vi "AuMT8852B Initial Carrier Extended Results Query.vi"(7 "Stage":T1(ring), 8 "error in (no error)":errorcluster, 11 "VISA session":refnum<visa-resource-name>) -> (0 "error out":errorcluster, 2 "error code":i32, 3 "VISA session out":refnum<visa-resource-name>, 4 "Results":T2 {"Max negative offset (kHz)" format="%.2f"; "Max positive offset (kHz)" format="%.2f"; "Test average offset (kHz)" format="%.2f"})   [LabVIEW 2017]
doc: "Anritsu MT8852B Bluetooth Tester\n\nReturns the results of the Initial Carrier test.\n\nINPUTS\nStage - results of the individual hopping stages of the test.\n\nOUTPUTS\nResults - measurements made during the test."
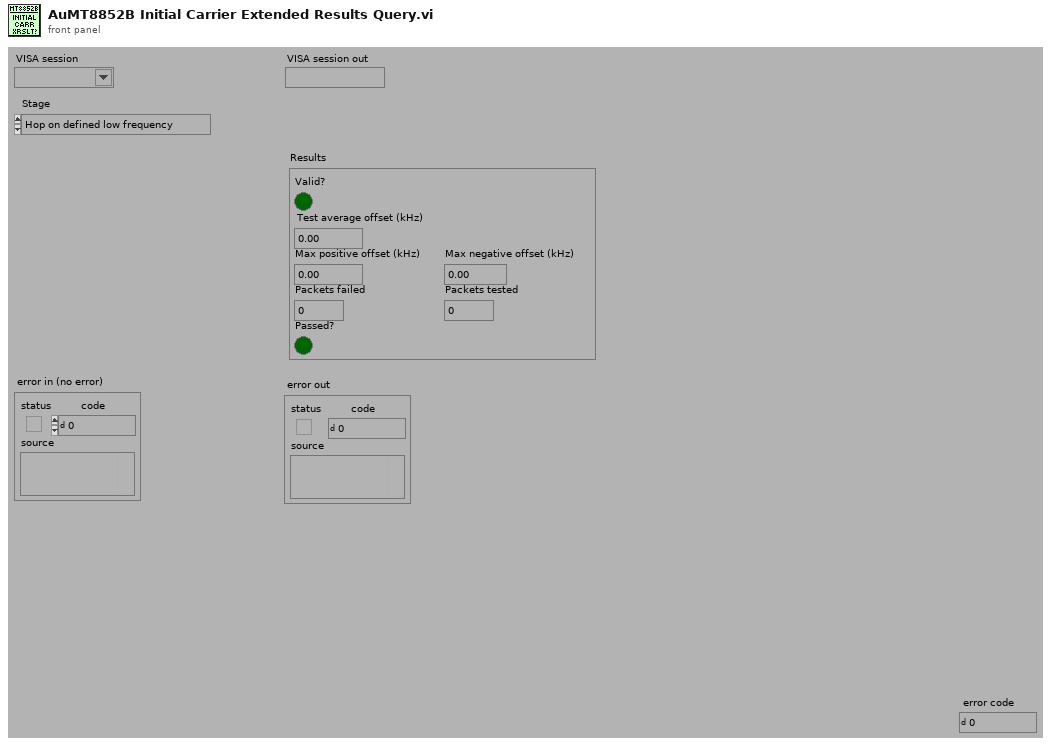
[diagram p1: front panel]
types:
  T1 = enum16{"Hop on defined low frequency", "Hop on defined medium frequency", "Hop on defined high frequency", "Hop on all channels", "Hop on any channels", "Hop off low frequency", "Hop off medium frequency", "Hop off high frequency"}
  T2 = cluster{"Valid?":bool, "Test average offset (kHz)":dbl, "Max positive offset (kHz)":dbl, "Max negative offset (kHz)":dbl, "Passed?":bool, "Packets failed":i32, "Packets tested":i32}
  T3 = enum16{"Simulate", "Range check", "Cache", "Query instrument status"}
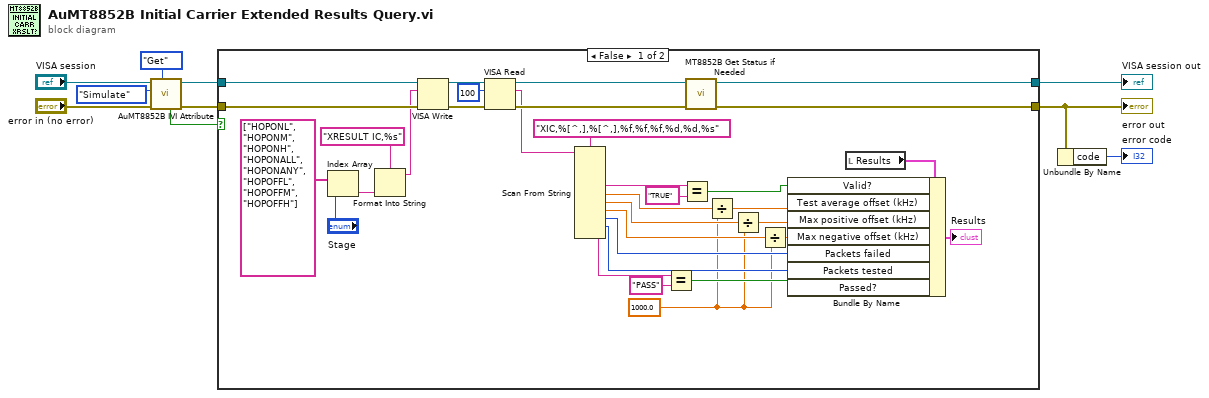
[diagram p0: block diagram]
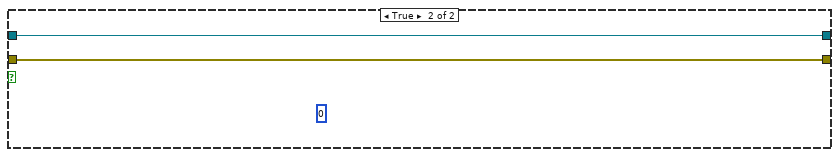
[diagram p2: hidden frame]
diagram:
  n1 = call <instrlib>:"AuMT8852B IVI Attribute.vi"("Set/Get (Set)"=enum16{"Set", "Get"}."Get", "error in (no error)"="error in (no error)", "Flag (Simulate)"=T3."Simulate", "VISA session"="VISA session") -> ("error out"=w7:errorcluster, "VISA session out"=w9:refnum<visa-resource-name>, "Value out"=w3:bool)  [unwired: 5 in]
  n2 = case shown="False" w3 {
    tunnel: [w33 w45] -> w10
    tunnel: [w32 w44] -> w1
    tunnel: w9 -> [w43 w45]
    tunnel: w7 -> [w42 w44]
    frame False {
      w11 = 1000.0 ("y")
      n3 = Index Array(array=string[] ["HOPONL", "HOPONM", "HOPONH", "HOPONALL", "HOPONANY", "HOPOFFL", "HOPOFFM", "HOPOFFH"], index="Stage") -> (element=w27:string)
      n4 = Format Into String(format string="XRESULT IC,%s" ("write buffer (\"\")"), w27) -> (resulting string=w19:string)  [unwired: 2 in, 1 out]
      n5 = VISA Write(VISA resource name=w43, write buffer=w19, error in (no error)=w42) -> (VISA resource name out=w41:refnum<visa-resource-name>, error out=w40:errorcluster)  [unwired: 1 out]
      n6 = VISA Read(VISA resource name=w41, byte count=u32 100 ("byte count (0)"), error in (no error)=w40) -> (VISA resource name out=w31:refnum<visa-resource-name>, read buffer=w18:string, error out=w30:errorcluster)  [unwired: 1 out]
      n7 = Scan From String(format string="XIC,%[^,],%[^,],%f,%f,%f,%d,%d,%s" ("Format String"), input string=w18) -> (output 2=w24:string, output 3=w12:dbl, output 4=w13:dbl, output 5=w17:dbl, output 6=w22:i32, output 7=w21:i32, output 8=w20:string)  [unwired: 11 in, 3 out]
      n8 = Equal?(x=w20, y="PASS") -> (x = y?=w29:bool)
      n9 = Equal?(x=w24, y="TRUE") -> (x = y?=w23:bool)
      n10 = call <instrlib>:"MT8852B Get Status if Needed.vi"("error in (no error)"=w30, "VISA session"=w31) -> ("error out"=w32:errorcluster, "VISA session out"=w33:refnum<visa-resource-name>)  [unwired: 8 in]
      n11 = Divide(x=w12, y=w11) -> (x/y=w15:dbl)
      n12 = Divide(x=w13, y=w11) -> (x/y=w16:dbl)
      n13 = Divide(x=w17, y=w11) -> (x/y=w14:dbl)
      n14 = local read "Results"() -> (w37:T2)
      n15 = Bundle By Name(cluster=w37, "Valid?"=w23, "Test average offset (kHz)"=w15, "Max positive offset (kHz)"=w16, "Max negative offset (kHz)"=w14, "Packets failed"=w22, "Packets tested"=w21, "Passed?"=w29) -> (→"Results":T2)
    }
    frame True {
      (unwired) u8 0
    }
  }
  "error out" <- w1
  "VISA session out" <- w10
  n16 = Unbundle By Name(w1) -> ("code"=→"error code":i32)
